vi "F Dwf Analog In Status Data.vi"(7 "cdData":i32, 8 "error in (no error)":errorcluster, 10 "idxChannel":i32, 11 "hdwf":i32) -> (0 "error out":errorcluster, 1 "rgdVoltData":dbl[](array[numeric]), 3 "function return":i32)   [LabVIEW 2019, in "Olasdwf.lvlib"]
doc: "DWFAPI int FDwfAnalogInStatusData(HDWF hdwf, int idxChannel, double *rgdVoltData, int cdData);"
uses:
  Olasdwf.lvlib
  Windows/System32/dwf.dll
panel:
  out "cdData 2":i32
  in  "rgdVoltData in":dbl[](array[numeric])
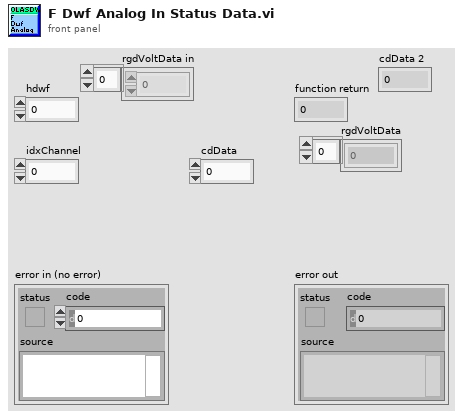
[diagram p1: front panel]
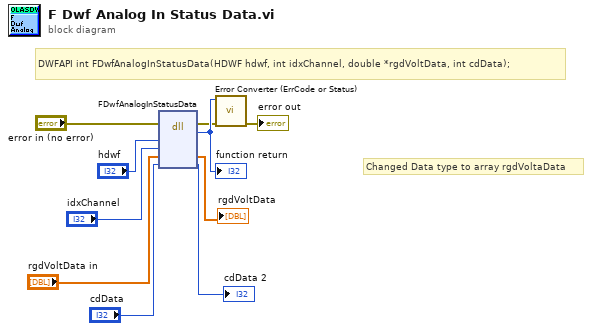
[diagram p0: block diagram]
diagram:
  # "Changed Data type to array rgdVoltaData"
  # "DWFAPI int FDwfAnalogInStatusData(HDWF hdwf, int idxChannel, double *rgdVoltData, int cdData);"
  n1 = dll-call lib="C:/Windows/System32/dwf.*" fn="FDwfAnalogInStatusData"(error in="error in (no error)", "hdwf"="hdwf", "idxChannel"="idxChannel", "rgdVoltData"="rgdVoltData in", "cdData"="cdData") -> (error out=w4:errorcluster, "return type"=w10:i32, "rgdVoltData"=→"rgdVoltData":dbl[], "cdData"=→"cdData 2":i32)  [unwired: 4 in, 1 out]
  "function return" <- w10
  n2 = call "Error Converter (ErrCode or Status).vi"("error in (no error)"=w4, "error code"=w10) -> ("error out"=→"error out":errorcluster)  [unwired: 9 in]
